vi "DataPointConv.vi"(10 "Stored Data":string) -> (2 "Data Points":dbl[][](array[numeric]))   [LabVIEW 2017]
panel:
  out "Numeric 2":dbl
  out "Stored Data 2":string
  out "Numeric":i32
  out "appended array":bool[](array[boolean])
  out "Block 14":string
  out "Block 6":string
  out "Block 1":string
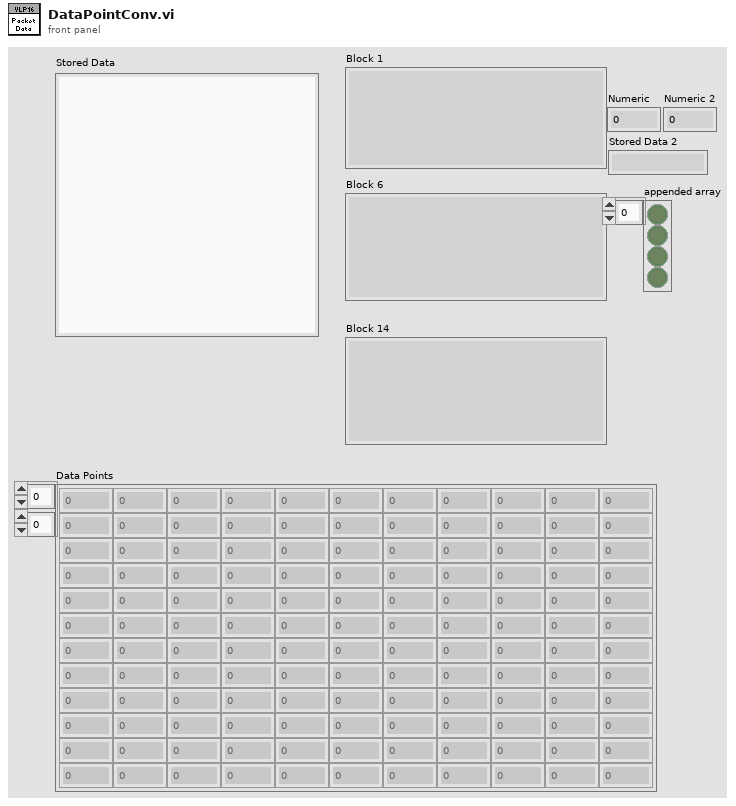
[diagram p1: front panel]
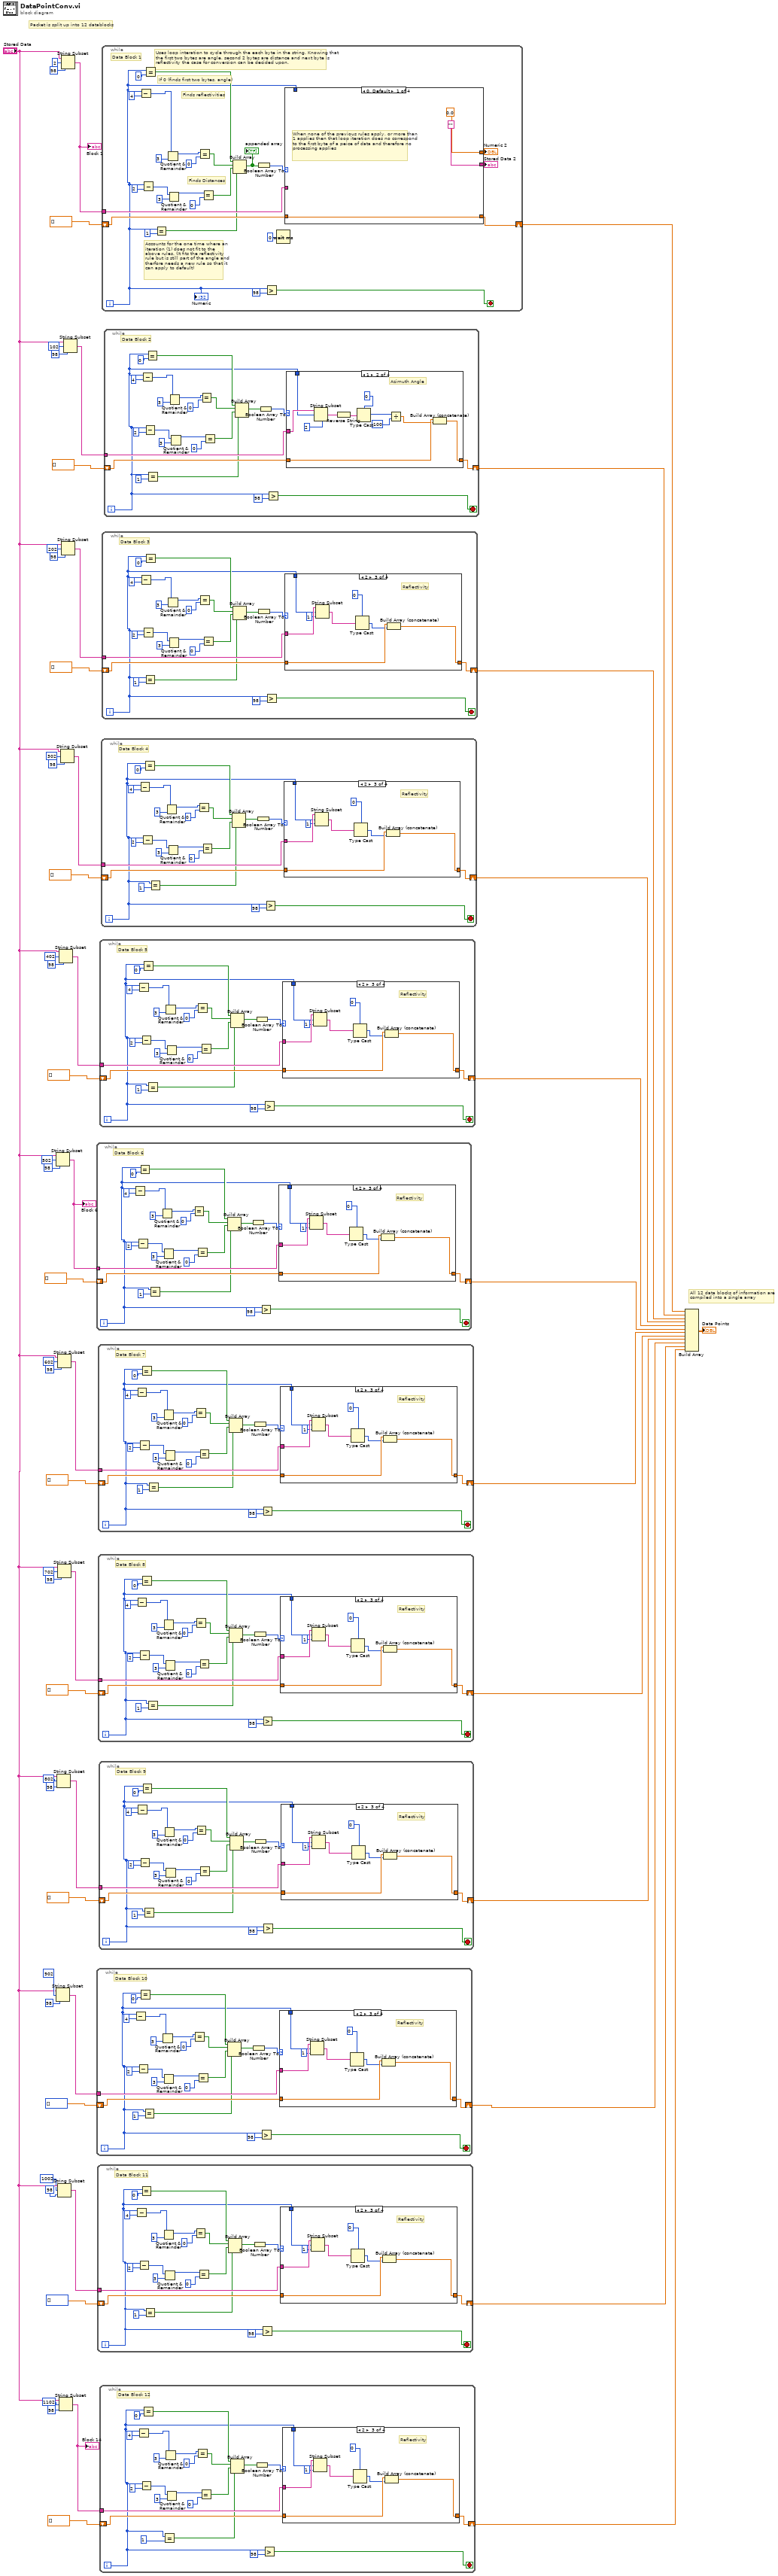
[diagram p0: block diagram]
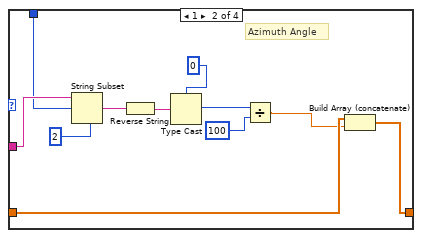
[diagram p3: hidden frame]
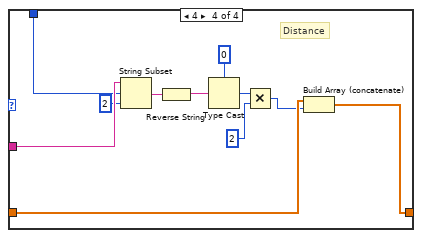
[diagram p4: hidden frame]
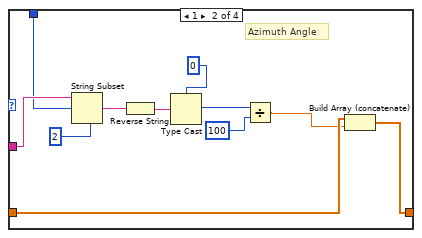
[diagram p6: hidden frame]
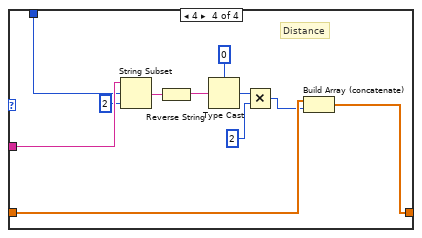
[diagram p7: hidden frame]
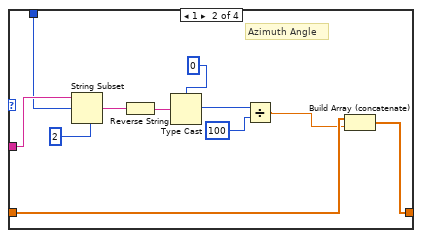
[diagram p9: hidden frame]
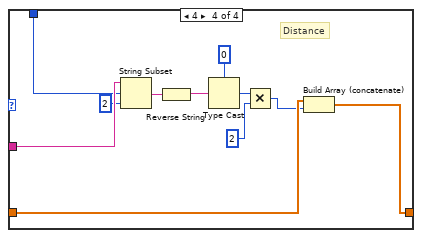
[diagram p10: hidden frame]
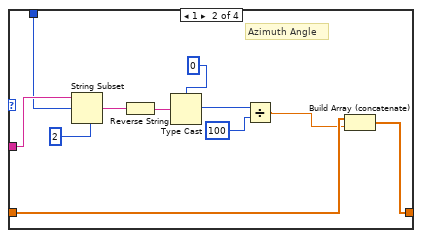
[diagram p12: hidden frame]
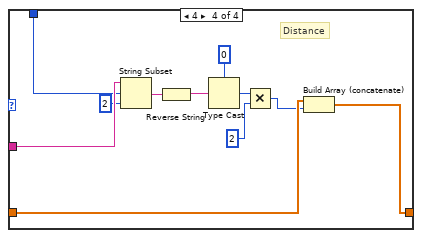
[diagram p13: hidden frame]
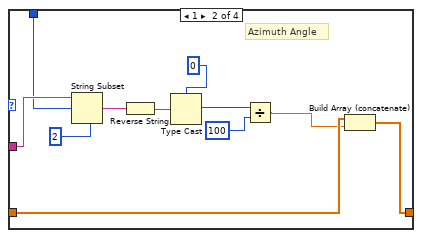
[diagram p15: hidden frame]
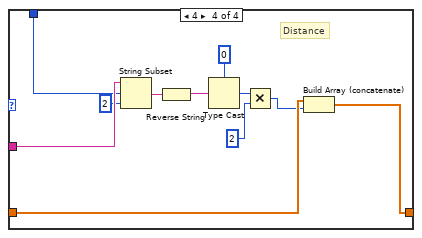
[diagram p16: hidden frame]
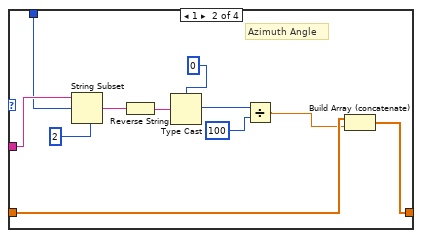
[diagram p18: hidden frame]
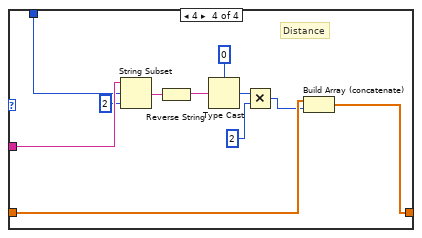
[diagram p19: hidden frame]
diagram:
  (unwired) u16[] []
  (unwired) u16[] []
  # "All 12 data blocks of information are\ncompiled into a single array"
  # "Packet is split up into 12 datablocks"
  n1 = String Subset(string="Stored Data", offset (0)=502, length (rest)=98 ("length (rest)")) -> (substring=w41:string)
  "Block 6" <- w41
  n2 = String Subset(string="Stored Data", offset (0)=902, length (rest)=98 ("length (rest)")) -> (substring=w24:string)
  n3 = String Subset(string="Stored Data", offset (0)=802, length (rest)=98 ("length (rest)")) -> (substring=w28:string)
  n4 = String Subset(string="Stored Data", offset (0)=602, length (rest)=98 ("length (rest)")) -> (substring=w36:string)
  n5 = String Subset(string="Stored Data", offset (0)=702, length (rest)=98 ("length (rest)")) -> (substring=w33:string)
  n6 = String Subset(string="Stored Data", offset (0)=1002, length (rest)=98 ("length (rest)")) -> (substring=w5:string)
  n7 = String Subset(string="Stored Data", offset (0)=402, length (rest)=98 ("length (rest)")) -> (substring=w44:string)
  n8 = String Subset(string="Stored Data", offset (0)=1102, length (rest)=98 ("length (rest)")) -> (substring=w20:string)
  "Block 14" <- w20
  n9 = String Subset(string="Stored Data", offset (0)=302, length (rest)=98 ("length (rest)")) -> (substring=w49:string)
  n10 = String Subset(string="Stored Data", offset (0)=2, length (rest)=98 ("length (rest)")) -> (substring=w60:string)
  "Block 1" <- w60
  n11 = String Subset(string="Stored Data", offset (0)=202, length (rest)=98 ("length (rest)")) -> (substring=w52:string)
  n12 = String Subset(string="Stored Data", offset (0)=102, length (rest)=98 ("length (rest)")) -> (substring=w57:string)
  n13 = while {
    tunnel: w41 -> [w86]
    shift-right: [w68] -> w11
    shift-left: dbl[] [] -> [w69]
    i -> [w64]
    stop <- w66 stop-if-true
    # "Data Block 6"
    n14 = Subtract(x=w64, y=4) -> (x-y=w72:i32)
    n15 = Subtract(x=w64, y=2) -> (x-y=w70:i32)
    n16 = Equal?(x=w64, y=0) -> (x = y?=w78:bool)
    n17 = Equal?(x=w64, y=1) -> (x = y?=w63:bool)
    n18 = Quotient & Remainder(x=w72, y=3) -> (x-y*floor(x/y)=w83:i32)  [unwired: 1 out]
    n19 = Quotient & Remainder(x=w70, y=3) -> (x-y*floor(x/y)=w79:i32)  [unwired: 1 out]
    n20 = Equal?(x=w83, y=0) -> (x = y?=w77:bool)
    n21 = Equal?(x=w79, y=0) -> (x = y?=w76:bool)
    n22 = Build Array(w78, w77, w76, w63) -> (w75:bool[])
    n23 = Boolean Array To Number(Boolean array=w75) -> (number=w74:u32)
    n24 = Greater?(x=w64, y=98) -> (0:w66:bool)
    n25 = case shown="2" w74 {
      tunnel: w86 -> [_ w98 w106 w117]
      tunnel: w64 -> [_ w97 w105 w116]
      tunnel: w69 -> [w87 w90 w101 w109]
      tunnel: [w87 w89 w99 w107] -> w68
      frame 0, Default {
      }
      frame 1 {
        # "Azimuth Angle"
        n26 = String Subset(string=w98, offset (0)=w97, length (rest)=2 ("length (rest)")) -> (substring=w95:string)
        n27 = Reverse String(1:w95) -> (0:w94:string)
        n28 = Type Cast(type=i16 0, x=w94) -> (*(type *) &x=w93:i16)
        n29 = Divide(x=w93, y=u16 100) -> (x/y=w88:dbl)
        n30 = Build Array (concatenate)(w90, w88) -> (w89:dbl[])
      }
      frame 2 {
        # "Reflectivity"
        n31 = String Subset(string=w106, offset (0)=w105, length (rest)=1 ("length (rest)")) -> (substring=w103:string)
        n32 = Type Cast(type=u8 0, x=w103) -> (*(type *) &x=w100:u8)
        n33 = Build Array (concatenate)(w101, w100) -> (w99:dbl[])
      }
      frame 4 {
        # "Distance"
        n34 = String Subset(string=w117, offset (0)=w116, length (rest)=2 ("length (rest)")) -> (substring=w114:string)
        n35 = Reverse String(1:w114) -> (0:w113:string)
        n36 = Type Cast(type=u16 0, x=w113) -> (*(type *) &x=w112:u16)
        n37 = Multiply(x=w112, y=u16 2) -> (x*y=w108:u16)
        n38 = Build Array (concatenate)(w109, w108) -> (w107:dbl[])
      }
    }
  }
  n39 = while {
    tunnel: w24 -> [w141]
    shift-right: [w123] -> w6
    shift-left: dbl[] [] -> [w124]
    i -> [w119]
    stop <- w121 stop-if-true
    # "Data Block 10"
    n40 = Subtract(x=w119, y=4) -> (x-y=w127:i32)
    n41 = Subtract(x=w119, y=2) -> (x-y=w125:i32)
    n42 = Equal?(x=w119, y=0) -> (x = y?=w133:bool)
    n43 = Equal?(x=w119, y=1) -> (x = y?=w118:bool)
    n44 = Quotient & Remainder(x=w127, y=3) -> (x-y*floor(x/y)=w138:i32)  [unwired: 1 out]
    n45 = Quotient & Remainder(x=w125, y=3) -> (x-y*floor(x/y)=w134:i32)  [unwired: 1 out]
    n46 = Equal?(x=w138, y=0) -> (x = y?=w132:bool)
    n47 = Equal?(x=w134, y=0) -> (x = y?=w131:bool)
    n48 = Build Array(w133, w132, w131, w118) -> (w130:bool[])
    n49 = Boolean Array To Number(Boolean array=w130) -> (number=w129:u32)
    n50 = Greater?(x=w119, y=98) -> (0:w121:bool)
    n51 = case shown="2" w129 {
      tunnel: w141 -> [_ w153 w161 w172]
      tunnel: w119 -> [_ w152 w160 w171]
      tunnel: w124 -> [w142 w145 w156 w164]
      tunnel: [w142 w144 w154 w162] -> w123
      frame 0, Default {
      }
      frame 1 {
        # "Azimuth Angle"
        n52 = String Subset(string=w153, offset (0)=w152, length (rest)=2 ("length (rest)")) -> (substring=w150:string)
        n53 = Reverse String(1:w150) -> (0:w149:string)
        n54 = Type Cast(type=i16 0, x=w149) -> (*(type *) &x=w148:i16)
        n55 = Divide(x=w148, y=u16 100) -> (x/y=w143:dbl)
        n56 = Build Array (concatenate)(w145, w143) -> (w144:dbl[])
      }
      frame 2 {
        # "Reflectivity"
        n57 = String Subset(string=w161, offset (0)=w160, length (rest)=1 ("length (rest)")) -> (substring=w158:string)
        n58 = Type Cast(type=u8 0, x=w158) -> (*(type *) &x=w155:u8)
        n59 = Build Array (concatenate)(w156, w155) -> (w154:dbl[])
      }
      frame 4 {
        # "Distance"
        n60 = String Subset(string=w172, offset (0)=w171, length (rest)=2 ("length (rest)")) -> (substring=w169:string)
        n61 = Reverse String(1:w169) -> (0:w168:string)
        n62 = Type Cast(type=u16 0, x=w168) -> (*(type *) &x=w167:u16)
        n63 = Multiply(x=w167, y=u16 2) -> (x*y=w163:u16)
        n64 = Build Array (concatenate)(w164, w163) -> (w162:dbl[])
      }
    }
  }
  n65 = while {
    tunnel: w5 -> [w196]
    shift-right: [w178] -> w2
    shift-left: dbl[] [] -> [w179]
    i -> [w174]
    stop <- w176 stop-if-true
    # "Data Block 11"
    n66 = Subtract(x=w174, y=4) -> (x-y=w182:i32)
    n67 = Subtract(x=w174, y=2) -> (x-y=w180:i32)
    n68 = Equal?(x=w174, y=0) -> (x = y?=w188:bool)
    n69 = Equal?(x=w174, y=1) -> (x = y?=w173:bool)
    n70 = Quotient & Remainder(x=w182, y=3) -> (x-y*floor(x/y)=w193:i32)  [unwired: 1 out]
    n71 = Quotient & Remainder(x=w180, y=3) -> (x-y*floor(x/y)=w189:i32)  [unwired: 1 out]
    n72 = Equal?(x=w193, y=0) -> (x = y?=w187:bool)
    n73 = Equal?(x=w189, y=0) -> (x = y?=w186:bool)
    n74 = Build Array(w188, w187, w186, w173) -> (w185:bool[])
    n75 = Boolean Array To Number(Boolean array=w185) -> (number=w184:u32)
    n76 = Greater?(x=w174, y=98) -> (0:w176:bool)
    n77 = case shown="2" w184 {
      tunnel: w196 -> [_ w208 w216 w227]
      tunnel: w174 -> [_ w207 w215 w226]
      tunnel: w179 -> [w197 w200 w211 w219]
      tunnel: [w197 w199 w209 w217] -> w178
      frame 0, Default {
      }
      frame 1 {
        # "Azimuth Angle"
        n78 = String Subset(string=w208, offset (0)=w207, length (rest)=2 ("length (rest)")) -> (substring=w205:string)
        n79 = Reverse String(1:w205) -> (0:w204:string)
        n80 = Type Cast(type=i16 0, x=w204) -> (*(type *) &x=w203:i16)
        n81 = Divide(x=w203, y=u16 100) -> (x/y=w198:dbl)
        n82 = Build Array (concatenate)(w200, w198) -> (w199:dbl[])
      }
      frame 2 {
        # "Reflectivity"
        n83 = String Subset(string=w216, offset (0)=w215, length (rest)=1 ("length (rest)")) -> (substring=w213:string)
        n84 = Type Cast(type=u8 0, x=w213) -> (*(type *) &x=w210:u8)
        n85 = Build Array (concatenate)(w211, w210) -> (w209:dbl[])
      }
      frame 4 {
        # "Distance"
        n86 = String Subset(string=w227, offset (0)=w226, length (rest)=2 ("length (rest)")) -> (substring=w224:string)
        n87 = Reverse String(1:w224) -> (0:w223:string)
        n88 = Type Cast(type=u16 0, x=w223) -> (*(type *) &x=w222:u16)
        n89 = Multiply(x=w222, y=u16 2) -> (x*y=w218:u16)
        n90 = Build Array (concatenate)(w219, w218) -> (w217:dbl[])
      }
    }
  }
  n91 = while {
    tunnel: w36 -> [w251]
    shift-right: [w233] -> w10
    shift-left: dbl[] [] -> [w234]
    i -> [w229]
    stop <- w231 stop-if-true
    # "Data Block 7"
    n92 = Subtract(x=w229, y=4) -> (x-y=w237:i32)
    n93 = Subtract(x=w229, y=2) -> (x-y=w235:i32)
    n94 = Equal?(x=w229, y=0) -> (x = y?=w243:bool)
    n95 = Equal?(x=w229, y=1) -> (x = y?=w228:bool)
    n96 = Quotient & Remainder(x=w237, y=3) -> (x-y*floor(x/y)=w248:i32)  [unwired: 1 out]
    n97 = Quotient & Remainder(x=w235, y=3) -> (x-y*floor(x/y)=w244:i32)  [unwired: 1 out]
    n98 = Equal?(x=w248, y=0) -> (x = y?=w242:bool)
    n99 = Equal?(x=w244, y=0) -> (x = y?=w241:bool)
    n100 = Build Array(w243, w242, w241, w228) -> (w240:bool[])
    n101 = Boolean Array To Number(Boolean array=w240) -> (number=w239:u32)
    n102 = Greater?(x=w229, y=98) -> (0:w231:bool)
    n103 = case shown="2" w239 {
      tunnel: w251 -> [_ w263 w271 w282]
      tunnel: w229 -> [_ w262 w270 w281]
      tunnel: w234 -> [w252 w255 w266 w274]
      tunnel: [w252 w254 w264 w272] -> w233
      frame 0, Default {
      }
      frame 1 {
        # "Azimuth Angle"
        n104 = String Subset(string=w263, offset (0)=w262, length (rest)=2 ("length (rest)")) -> (substring=w260:string)
        n105 = Reverse String(1:w260) -> (0:w259:string)
        n106 = Type Cast(type=i16 0, x=w259) -> (*(type *) &x=w258:i16)
        n107 = Divide(x=w258, y=u16 100) -> (x/y=w253:dbl)
        n108 = Build Array (concatenate)(w255, w253) -> (w254:dbl[])
      }
      frame 2 {
        # "Reflectivity"
        n109 = String Subset(string=w271, offset (0)=w270, length (rest)=1 ("length (rest)")) -> (substring=w268:string)
        n110 = Type Cast(type=u8 0, x=w268) -> (*(type *) &x=w265:u8)
        n111 = Build Array (concatenate)(w266, w265) -> (w264:dbl[])
      }
      frame 4 {
        # "Distance"
        n112 = String Subset(string=w282, offset (0)=w281, length (rest)=2 ("length (rest)")) -> (substring=w279:string)
        n113 = Reverse String(1:w279) -> (0:w278:string)
        n114 = Type Cast(type=u16 0, x=w278) -> (*(type *) &x=w277:u16)
        n115 = Multiply(x=w277, y=u16 2) -> (x*y=w273:u16)
        n116 = Build Array (concatenate)(w274, w273) -> (w272:dbl[])
      }
    }
  }
  n117 = while {
    tunnel: w33 -> [w306]
    shift-right: [w288] -> w9
    shift-left: dbl[] [] -> [w289]
    i -> [w284]
    stop <- w286 stop-if-true
    # "Data Block 8"
    n118 = Subtract(x=w284, y=4) -> (x-y=w292:i32)
    n119 = Subtract(x=w284, y=2) -> (x-y=w290:i32)
    n120 = Equal?(x=w284, y=0) -> (x = y?=w298:bool)
    n121 = Equal?(x=w284, y=1) -> (x = y?=w283:bool)
    n122 = Quotient & Remainder(x=w292, y=3) -> (x-y*floor(x/y)=w303:i32)  [unwired: 1 out]
    n123 = Quotient & Remainder(x=w290, y=3) -> (x-y*floor(x/y)=w299:i32)  [unwired: 1 out]
    n124 = Equal?(x=w303, y=0) -> (x = y?=w297:bool)
    n125 = Equal?(x=w299, y=0) -> (x = y?=w296:bool)
    n126 = Build Array(w298, w297, w296, w283) -> (w295:bool[])
    n127 = Boolean Array To Number(Boolean array=w295) -> (number=w294:u32)
    n128 = Greater?(x=w284, y=98) -> (0:w286:bool)
    n129 = case shown="2" w294 {
      tunnel: w306 -> [_ w318 w326 w337]
      tunnel: w284 -> [_ w317 w325 w336]
      tunnel: w289 -> [w307 w310 w321 w329]
      tunnel: [w307 w309 w319 w327] -> w288
      frame 0, Default {
      }
      frame 1 {
        # "Azimuth Angle"
        n130 = String Subset(string=w318, offset (0)=w317, length (rest)=2 ("length (rest)")) -> (substring=w315:string)
        n131 = Reverse String(1:w315) -> (0:w314:string)
        n132 = Type Cast(type=i16 0, x=w314) -> (*(type *) &x=w313:i16)
        n133 = Divide(x=w313, y=u16 100) -> (x/y=w308:dbl)
        n134 = Build Array (concatenate)(w310, w308) -> (w309:dbl[])
      }
      frame 2 {
        # "Reflectivity"
        n135 = String Subset(string=w326, offset (0)=w325, length (rest)=1 ("length (rest)")) -> (substring=w323:string)
        n136 = Type Cast(type=u8 0, x=w323) -> (*(type *) &x=w320:u8)
        n137 = Build Array (concatenate)(w321, w320) -> (w319:dbl[])
      }
      frame 4 {
        # "Distance"
        n138 = String Subset(string=w337, offset (0)=w336, length (rest)=2 ("length (rest)")) -> (substring=w334:string)
        n139 = Reverse String(1:w334) -> (0:w333:string)
        n140 = Type Cast(type=u16 0, x=w333) -> (*(type *) &x=w332:u16)
        n141 = Multiply(x=w332, y=u16 2) -> (x*y=w328:u16)
        n142 = Build Array (concatenate)(w329, w328) -> (w327:dbl[])
      }
    }
  }
  n143 = while {
    tunnel: w28 -> [w361]
    shift-right: [w343] -> w8
    shift-left: dbl[] [] -> [w344]
    i -> [w339]
    stop <- w341 stop-if-true
    # "Data Block 9"
    n144 = Subtract(x=w339, y=4) -> (x-y=w347:i32)
    n145 = Subtract(x=w339, y=2) -> (x-y=w345:i32)
    n146 = Equal?(x=w339, y=0) -> (x = y?=w353:bool)
    n147 = Equal?(x=w339, y=1) -> (x = y?=w338:bool)
    n148 = Quotient & Remainder(x=w347, y=3) -> (x-y*floor(x/y)=w358:i32)  [unwired: 1 out]
    n149 = Quotient & Remainder(x=w345, y=3) -> (x-y*floor(x/y)=w354:i32)  [unwired: 1 out]
    n150 = Equal?(x=w358, y=0) -> (x = y?=w352:bool)
    n151 = Equal?(x=w354, y=0) -> (x = y?=w351:bool)
    n152 = Build Array(w353, w352, w351, w338) -> (w350:bool[])
    n153 = Boolean Array To Number(Boolean array=w350) -> (number=w349:u32)
    n154 = Greater?(x=w339, y=98) -> (0:w341:bool)
    n155 = case shown="2" w349 {
      tunnel: w361 -> [_ w373 w381 w392]
      tunnel: w339 -> [_ w372 w380 w391]
      tunnel: w344 -> [w362 w365 w376 w384]
      tunnel: [w362 w364 w374 w382] -> w343
      frame 0, Default {
      }
      frame 1 {
        # "Azimuth Angle"
        n156 = String Subset(string=w373, offset (0)=w372, length (rest)=2 ("length (rest)")) -> (substring=w370:string)
        n157 = Reverse String(1:w370) -> (0:w369:string)
        n158 = Type Cast(type=i16 0, x=w369) -> (*(type *) &x=w368:i16)
        n159 = Divide(x=w368, y=u16 100) -> (x/y=w363:dbl)
        n160 = Build Array (concatenate)(w365, w363) -> (w364:dbl[])
      }
      frame 2 {
        # "Reflectivity"
        n161 = String Subset(string=w381, offset (0)=w380, length (rest)=1 ("length (rest)")) -> (substring=w378:string)
        n162 = Type Cast(type=u8 0, x=w378) -> (*(type *) &x=w375:u8)
        n163 = Build Array (concatenate)(w376, w375) -> (w374:dbl[])
      }
      frame 4 {
        # "Distance"
        n164 = String Subset(string=w392, offset (0)=w391, length (rest)=2 ("length (rest)")) -> (substring=w389:string)
        n165 = Reverse String(1:w389) -> (0:w388:string)
        n166 = Type Cast(type=u16 0, x=w388) -> (*(type *) &x=w387:u16)
        n167 = Multiply(x=w387, y=u16 2) -> (x*y=w383:u16)
        n168 = Build Array (concatenate)(w384, w383) -> (w382:dbl[])
      }
    }
  }
  n169 = while {
    tunnel: w44 -> [w416]
    shift-right: [w398] -> w12
    shift-left: dbl[] [] -> [w399]
    i -> [w394]
    stop <- w396 stop-if-true
    # "Data Block 5"
    n170 = Subtract(x=w394, y=4) -> (x-y=w402:i32)
    n171 = Subtract(x=w394, y=2) -> (x-y=w400:i32)
    n172 = Equal?(x=w394, y=0) -> (x = y?=w408:bool)
    n173 = Equal?(x=w394, y=1) -> (x = y?=w393:bool)
    n174 = Quotient & Remainder(x=w402, y=3) -> (x-y*floor(x/y)=w413:i32)  [unwired: 1 out]
    n175 = Quotient & Remainder(x=w400, y=3) -> (x-y*floor(x/y)=w409:i32)  [unwired: 1 out]
    n176 = Equal?(x=w413, y=0) -> (x = y?=w407:bool)
    n177 = Equal?(x=w409, y=0) -> (x = y?=w406:bool)
    n178 = Build Array(w408, w407, w406, w393) -> (w405:bool[])
    n179 = Boolean Array To Number(Boolean array=w405) -> (number=w404:u32)
    n180 = Greater?(x=w394, y=98) -> (0:w396:bool)
    n181 = case shown="2" w404 {
      tunnel: w416 -> [_ w428 w436 w447]
      tunnel: w394 -> [_ w427 w435 w446]
      tunnel: w399 -> [w417 w420 w431 w439]
      tunnel: [w417 w419 w429 w437] -> w398
      frame 0, Default {
      }
      frame 1 {
        # "Azimuth Angle"
        n182 = String Subset(string=w428, offset (0)=w427, length (rest)=2 ("length (rest)")) -> (substring=w425:string)
        n183 = Reverse String(1:w425) -> (0:w424:string)
        n184 = Type Cast(type=i16 0, x=w424) -> (*(type *) &x=w423:i16)
        n185 = Divide(x=w423, y=u16 100) -> (x/y=w418:dbl)
        n186 = Build Array (concatenate)(w420, w418) -> (w419:dbl[])
      }
      frame 2 {
        # "Reflectivity"
        n187 = String Subset(string=w436, offset (0)=w435, length (rest)=1 ("length (rest)")) -> (substring=w433:string)
        n188 = Type Cast(type=u8 0, x=w433) -> (*(type *) &x=w430:u8)
        n189 = Build Array (concatenate)(w431, w430) -> (w429:dbl[])
      }
      frame 4 {
        # "Distance"
        n190 = String Subset(string=w447, offset (0)=w446, length (rest)=2 ("length (rest)")) -> (substring=w444:string)
        n191 = Reverse String(1:w444) -> (0:w443:string)
        n192 = Type Cast(type=u16 0, x=w443) -> (*(type *) &x=w442:u16)
        n193 = Multiply(x=w442, y=u16 2) -> (x*y=w438:u16)
        n194 = Build Array (concatenate)(w439, w438) -> (w437:dbl[])
      }
    }
  }
  n195 = while {
    tunnel: w20 -> [w471]
    shift-right: [w453] -> w7
    shift-left: dbl[] [] -> [w454]
    i -> [w449]
    stop <- w451 stop-if-true
    # "Data Block 12"
    n196 = Subtract(x=w449, y=4) -> (x-y=w457:i32)
    n197 = Subtract(x=w449, y=2) -> (x-y=w455:i32)
    n198 = Equal?(x=w449, y=0) -> (x = y?=w463:bool)
    n199 = Equal?(x=w449, y=1) -> (x = y?=w448:bool)
    n200 = Quotient & Remainder(x=w457, y=3) -> (x-y*floor(x/y)=w468:i32)  [unwired: 1 out]
    n201 = Quotient & Remainder(x=w455, y=3) -> (x-y*floor(x/y)=w464:i32)  [unwired: 1 out]
    n202 = Equal?(x=w468, y=0) -> (x = y?=w462:bool)
    n203 = Equal?(x=w464, y=0) -> (x = y?=w461:bool)
    n204 = Build Array(w463, w462, w461, w448) -> (w460:bool[])
    n205 = Boolean Array To Number(Boolean array=w460) -> (number=w459:u32)
    n206 = Greater?(x=w449, y=98) -> (0:w451:bool)
    n207 = case shown="2" w459 {
      tunnel: w471 -> [_ w483 w491 w502]
      tunnel: w449 -> [_ w482 w490 w501]
      tunnel: w454 -> [w472 w475 w486 w494]
      tunnel: [w472 w474 w484 w492] -> w453
      frame 0, Default {
      }
      frame 1 {
        # "Azimuth Angle"
        n208 = String Subset(string=w483, offset (0)=w482, length (rest)=2 ("length (rest)")) -> (substring=w480:string)
        n209 = Reverse String(1:w480) -> (0:w479:string)
        n210 = Type Cast(type=i16 0, x=w479) -> (*(type *) &x=w478:i16)
        n211 = Divide(x=w478, y=u16 100) -> (x/y=w473:dbl)
        n212 = Build Array (concatenate)(w475, w473) -> (w474:dbl[])
      }
      frame 2 {
        # "Reflectivity"
        n213 = String Subset(string=w491, offset (0)=w490, length (rest)=1 ("length (rest)")) -> (substring=w488:string)
        n214 = Type Cast(type=u8 0, x=w488) -> (*(type *) &x=w485:u8)
        n215 = Build Array (concatenate)(w486, w485) -> (w484:dbl[])
      }
      frame 4 {
        # "Distance"
        n216 = String Subset(string=w502, offset (0)=w501, length (rest)=2 ("length (rest)")) -> (substring=w499:string)
        n217 = Reverse String(1:w499) -> (0:w498:string)
        n218 = Type Cast(type=u16 0, x=w498) -> (*(type *) &x=w497:u16)
        n219 = Multiply(x=w497, y=u16 2) -> (x*y=w493:u16)
        n220 = Build Array (concatenate)(w494, w493) -> (w492:dbl[])
      }
    }
  }
  n221 = while {
    tunnel: w49 -> [w526]
    shift-right: [w508] -> w13
    shift-left: dbl[] [] -> [w509]
    i -> [w504]
    stop <- w506 stop-if-true
    # "Data Block 4"
    n222 = Subtract(x=w504, y=4) -> (x-y=w512:i32)
    n223 = Subtract(x=w504, y=2) -> (x-y=w510:i32)
    n224 = Equal?(x=w504, y=0) -> (x = y?=w518:bool)
    n225 = Equal?(x=w504, y=1) -> (x = y?=w503:bool)
    n226 = Quotient & Remainder(x=w512, y=3) -> (x-y*floor(x/y)=w523:i32)  [unwired: 1 out]
    n227 = Quotient & Remainder(x=w510, y=3) -> (x-y*floor(x/y)=w519:i32)  [unwired: 1 out]
    n228 = Equal?(x=w523, y=0) -> (x = y?=w517:bool)
    n229 = Equal?(x=w519, y=0) -> (x = y?=w516:bool)
    n230 = Build Array(w518, w517, w516, w503) -> (w515:bool[])
    n231 = Boolean Array To Number(Boolean array=w515) -> (number=w514:u32)
    n232 = Greater?(x=w504, y=98) -> (0:w506:bool)
    n233 = case shown="2" w514 {
      tunnel: w526 -> [_ w538 w546 w557]
      tunnel: w504 -> [_ w537 w545 w556]
      tunnel: w509 -> [w527 w530 w541 w549]
      tunnel: [w527 w529 w539 w547] -> w508
      frame 0, Default {
      }
      frame 1 {
        # "Azimuth Angle"
        n234 = String Subset(string=w538, offset (0)=w537, length (rest)=2 ("length (rest)")) -> (substring=w535:string)
        n235 = Reverse String(1:w535) -> (0:w534:string)
        n236 = Type Cast(type=i16 0, x=w534) -> (*(type *) &x=w533:i16)
        n237 = Divide(x=w533, y=u16 100) -> (x/y=w528:dbl)
        n238 = Build Array (concatenate)(w530, w528) -> (w529:dbl[])
      }
      frame 2 {
        # "Reflectivity"
        n239 = String Subset(string=w546, offset (0)=w545, length (rest)=1 ("length (rest)")) -> (substring=w543:string)
        n240 = Type Cast(type=u8 0, x=w543) -> (*(type *) &x=w540:u8)
        n241 = Build Array (concatenate)(w541, w540) -> (w539:dbl[])
      }
      frame 4 {
        # "Distance"
        n242 = String Subset(string=w557, offset (0)=w556, length (rest)=2 ("length (rest)")) -> (substring=w554:string)
        n243 = Reverse String(1:w554) -> (0:w553:string)
        n244 = Type Cast(type=u16 0, x=w553) -> (*(type *) &x=w552:u16)
        n245 = Multiply(x=w552, y=u16 2) -> (x*y=w548:u16)
        n246 = Build Array (concatenate)(w549, w548) -> (w547:dbl[])
      }
    }
  }
  n247 = while {
    tunnel: w60 -> [w584]
    shift-right: [w566] -> w16
    shift-left: dbl[] [] -> [w567]
    i -> [w563]
    stop <- w564 stop-if-true
    # "Accounts for the one time where an iteration (1) does not fit to the above rules. (It fits the reflectivity rule but is still part of the angle and therfore needs a new rule so that it can apply to default)"
    # "Finds Distances"
    # "Finds reflectivities"
    # "If 0 (finds first two bytes, angle)"
    # "Uses loop interation to cycle through the each byte in the string. Knowing that the first two bytes are angle, second 2 bytes are distance and next byte is reflectivity the case for conversion can be decided upon."
    # "Data Block 1"
    n248 = Subtract(x=w563, y=4) -> (x-y=w570:i32)
    n249 = Subtract(x=w563, y=2) -> (x-y=w568:i32)
    n250 = Equal?(x=w563, y=0) -> (x = y?=w576:bool)
    n251 = Equal?(x=w563, y=1) -> (x = y?=w561:bool)
    n252 = Quotient & Remainder(x=w570, y=3) -> (x-y*floor(x/y)=w581:i32)  [unwired: 1 out]
    n253 = Quotient & Remainder(x=w568, y=3) -> (x-y*floor(x/y)=w577:i32)  [unwired: 1 out]
    n254 = Equal?(x=w581, y=0) -> (x = y?=w575:bool)
    n255 = Equal?(x=w577, y=0) -> (x = y?=w574:bool)
    n256 = Build Array(w576, w575, w574, w561) -> (w573:bool[])
    "appended array" <- w573
    n257 = Boolean Array To Number(Boolean array=w573) -> (number=w572:u32)
    n258 = Greater?(x=w563, y=98) -> (0:w564:bool)
    n259 = Wait (ms)(milliseconds to wait=u32 0) -> ()  [unwired: 1 out]
    n260 = case shown="0, Default" w572 {
      tunnel: w584 -> [_ w598 w606 w617]
      tunnel: w563 -> [_ w597 w605 w616]
      tunnel: w567 -> [w587 w592 w602 w611]
      tunnel: [w587 w591 w601 w610] -> w566
      tunnel: [0.0 w590 w600 w609] -> w558
      tunnel: ["" w588 w599 w607] -> w559
      frame 0, Default {
        # "When none of the previous rules apply, or more than 1 applies then that loop iteration does no correspond to the first byte of a peice of data and therefore no processing applies"
      }
      frame 1 {
        # "When the first rule applies than it is the beginning of the datablock and the next 2 bytes are taken and converted into a firing angle. (Conversion instructions in VLP-16 Manual)"
        # "Azimuth Angle"
        n261 = String Subset(string=w598, offset (0)=w597, length (rest)=2 ("length (rest)")) -> (substring=w588:string)
        n262 = Reverse String(1:w588) -> (0:w589:string)
        n263 = Type Cast(type=i16 0, x=w589) -> (*(type *) &x=w595:i16)
        n264 = Divide(x=w595, y=u16 100) -> (x/y=w590:dbl)
        n265 = Build Array (concatenate)(w592, w590) -> (w591:dbl[])
      }
      frame 2 {
        # "When the 2nd rule applies than ir corresponds to the beginning byte of\nreflectivity data. The single byte is taken and converted into a reflectivity \n(simply converted to a decimal number)"
        # "Reflectivity"
        n266 = String Subset(string=w606, offset (0)=w605, length (rest)=1 ("length (rest)")) -> (substring=w599:string)
        n267 = Type Cast(type=u8 0, x=w599) -> (*(type *) &x=w600:u8)
        n268 = Build Array (concatenate)(w602, w600) -> (w601:dbl[])
      }
      frame 4 {
        # "When the 3rd rule applies then it corresponds to the beginning of 2 \nbytes of distance data. The two bytes are taken and converted to a \ndistance in mm (conversion instructions in VLP-16 manual)"
        # "Distance"
        n269 = String Subset(string=w617, offset (0)=w616, length (rest)=2 ("length (rest)")) -> (substring=w607:string)
        n270 = Reverse String(1:w607) -> (0:w608:string)
        n271 = Type Cast(type=u16 0, x=w608) -> (*(type *) &x=w614:u16)
        n272 = Multiply(x=w614, y=u16 2) -> (x*y=w609:u16)
        n273 = Build Array (concatenate)(w611, w609) -> (w610:dbl[])
      }
    }
    "Stored Data 2" <- w559
    "Numeric 2" <- w558
    "Numeric" <- w563
  }
  n274 = while {
    tunnel: w52 -> [w641]
    shift-right: [w623] -> w14
    shift-left: dbl[] [] -> [w624]
    i -> [w620]
    stop <- w621 stop-if-true
    # "Data Block 3"
    n275 = Subtract(x=w620, y=4) -> (x-y=w627:i32)
    n276 = Subtract(x=w620, y=2) -> (x-y=w625:i32)
    n277 = Equal?(x=w620, y=1) -> (x = y?=w618:bool)
    n278 = Equal?(x=w620, y=0) -> (x = y?=w633:bool)
    n279 = Quotient & Remainder(x=w627, y=3) -> (x-y*floor(x/y)=w638:i32)  [unwired: 1 out]
    n280 = Quotient & Remainder(x=w625, y=3) -> (x-y*floor(x/y)=w634:i32)  [unwired: 1 out]
    n281 = Equal?(x=w638, y=0) -> (x = y?=w632:bool)
    n282 = Equal?(x=w634, y=0) -> (x = y?=w631:bool)
    n283 = Build Array(w633, w632, w631, w618) -> (w630:bool[])
    n284 = Boolean Array To Number(Boolean array=w630) -> (number=w629:u32)
    n285 = Greater?(x=w620, y=98) -> (0:w621:bool)
    n286 = case shown="2" w629 {
      tunnel: w641 -> [_ w653 w661 w672]
      tunnel: w620 -> [_ w652 w660 w671]
      tunnel: w624 -> [w642 w645 w656 w664]
      tunnel: [w642 w644 w654 w662] -> w623
      frame 0, Default {
      }
      frame 1 {
        # "Azimuth Angle"
        n287 = String Subset(string=w653, offset (0)=w652, length (rest)=2 ("length (rest)")) -> (substring=w650:string)
        n288 = Reverse String(1:w650) -> (0:w649:string)
        n289 = Type Cast(type=i16 0, x=w649) -> (*(type *) &x=w648:i16)
        n290 = Divide(x=w648, y=u16 100) -> (x/y=w643:dbl)
        n291 = Build Array (concatenate)(w645, w643) -> (w644:dbl[])
      }
      frame 2 {
        # "Reflectivity"
        n292 = String Subset(string=w661, offset (0)=w660, length (rest)=1 ("length (rest)")) -> (substring=w658:string)
        n293 = Type Cast(type=u8 0, x=w658) -> (*(type *) &x=w655:u8)
        n294 = Build Array (concatenate)(w656, w655) -> (w654:dbl[])
      }
      frame 4 {
        # "Distance"
        n295 = String Subset(string=w672, offset (0)=w671, length (rest)=2 ("length (rest)")) -> (substring=w669:string)
        n296 = Reverse String(1:w669) -> (0:w668:string)
        n297 = Type Cast(type=u16 0, x=w668) -> (*(type *) &x=w667:u16)
        n298 = Multiply(x=w667, y=u16 2) -> (x*y=w663:u16)
        n299 = Build Array (concatenate)(w664, w663) -> (w662:dbl[])
      }
    }
  }
  n300 = while {
    tunnel: w57 -> [w696]
    shift-right: [w678] -> w15
    shift-left: dbl[] [] -> [w679]
    i -> [w675]
    stop <- w676 stop-if-true
    # "Data Block 2"
    n301 = Subtract(x=w675, y=4) -> (x-y=w682:i32)
    n302 = Subtract(x=w675, y=2) -> (x-y=w680:i32)
    n303 = Equal?(x=w675, y=0) -> (x = y?=w688:bool)
    n304 = Equal?(x=w675, y=1) -> (x = y?=w673:bool)
    n305 = Quotient & Remainder(x=w682, y=3) -> (x-y*floor(x/y)=w693:i32)  [unwired: 1 out]
    n306 = Quotient & Remainder(x=w680, y=3) -> (x-y*floor(x/y)=w689:i32)  [unwired: 1 out]
    n307 = Equal?(x=w693, y=0) -> (x = y?=w687:bool)
    n308 = Equal?(x=w689, y=0) -> (x = y?=w686:bool)
    n309 = Build Array(w688, w687, w686, w673) -> (w685:bool[])
    n310 = Boolean Array To Number(Boolean array=w685) -> (number=w684:u32)
    n311 = Greater?(x=w675, y=98) -> (0:w676:bool)
    n312 = case shown="1" w684 {
      tunnel: w696 -> [_ w708 w716 w727]
      tunnel: w675 -> [_ w707 w715 w726]
      tunnel: w679 -> [w697 w700 w711 w719]
      tunnel: [w697 w699 w709 w717] -> w678
      frame 0, Default {
      }
      frame 1 {
        # "Azimuth Angle"
        n313 = String Subset(string=w708, offset (0)=w707, length (rest)=2 ("length (rest)")) -> (substring=w705:string)
        n314 = Reverse String(1:w705) -> (0:w704:string)
        n315 = Type Cast(type=i16 0, x=w704) -> (*(type *) &x=w703:i16)
        n316 = Divide(x=w703, y=u16 100) -> (x/y=w698:dbl)
        n317 = Build Array (concatenate)(w700, w698) -> (w699:dbl[])
      }
      frame 2 {
        # "Reflectivity"
        n318 = String Subset(string=w716, offset (0)=w715, length (rest)=1 ("length (rest)")) -> (substring=w713:string)
        n319 = Type Cast(type=u8 0, x=w713) -> (*(type *) &x=w710:u8)
        n320 = Build Array (concatenate)(w711, w710) -> (w709:dbl[])
      }
      frame 4 {
        # "Distance"
        n321 = String Subset(string=w727, offset (0)=w726, length (rest)=2 ("length (rest)")) -> (substring=w724:string)
        n322 = Reverse String(1:w724) -> (0:w723:string)
        n323 = Type Cast(type=u16 0, x=w723) -> (*(type *) &x=w722:u16)
        n324 = Multiply(x=w722, y=u16 2) -> (x*y=w718:u16)
        n325 = Build Array (concatenate)(w719, w718) -> (w717:dbl[])
      }
    }
  }
  n326 = Build Array(w16, w15, w14, w13, w12, w11, w10, w9, w8, w6, w2, w7) -> (→"Data Points":dbl[][])
